vi "MeasureFrequencySourceSelect.vi"(1 "Signal Type Select":u16(ring) items=["1Mhz", "1MHz MONITOR PLUG", "DSMP", "DSMP MONITOR PLUG", "RP", "RP MONITOR PLUG", "MP", "MP MONITOR PLUG", "EEP 1.2 Sec", "EEP MONITOR PLUG", "SMP DIFF", "SMP MONITOR PLUG", "SMP Open Collector"]) -> (0 "Numeric":i32 format="%.0x")   [LabVIEW 2013]
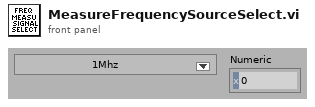
[diagram p1: front panel]
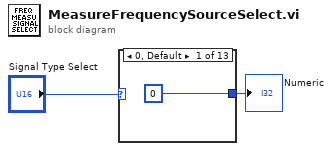
[diagram p0: block diagram]
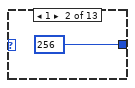
[diagram p2: hidden frame]
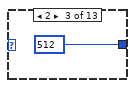
[diagram p3: hidden frame]
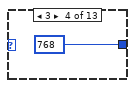
[diagram p4: hidden frame]
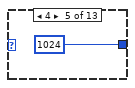
[diagram p5: hidden frame]
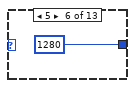
[diagram p6: hidden frame]
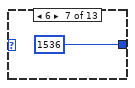
[diagram p7: hidden frame]
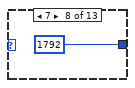
[diagram p8: hidden frame]
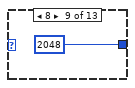
[diagram p9: hidden frame]
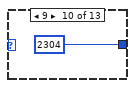
[diagram p10: hidden frame]
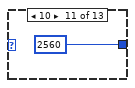
[diagram p11: hidden frame]
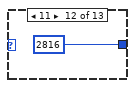
[diagram p12: hidden frame]
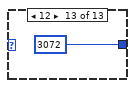
[diagram p13: hidden frame]
diagram:
  n1 = case shown="0, Default" "Signal Type Select" {
    tunnel: [0 256 512 768 1024 1280 1536 1792 2048 2304 2560 2816 3072] -> w2
    frame 0, Default {
    }
    frame 1 {
    }
    frame 2 {
    }
    frame 3 {
    }
    frame 4 {
    }
    frame 5 {
    }
    frame 6 {
    }
    frame 7 {
    }
    frame 8 {
    }
    frame 9 {
    }
    frame 10 {
    }
    frame 11 {
    }
    frame 12 {
    }
  }
  "Numeric" <- w2
